vi "Exist Section.vi"(10 "sections":string[](array[string]), 11 "info data":string) -> (1 "exist":bool, 2 "after end of section":string, 3 "before end of section":string)   [LabVIEW 2013, in "infolib.lvlib"]
doc: "Checks if sections structure exists, if so divides string before the end of least significant section."
uses:
  infolib.lvlib
  <vilib>/regexp/Match Regular Expression.xnode
panel:
  out "regexp":string
  # "testing string: (put \"1\" and \"2\" into section names)"
  # "blfdablad\n#startsection:: 1\njfkdla\n#startsection:: 2\ngroup2group2\n\t  \t#endsection:: 2\njdfkls\n#endsection:: 1\njfdklajfkdl"
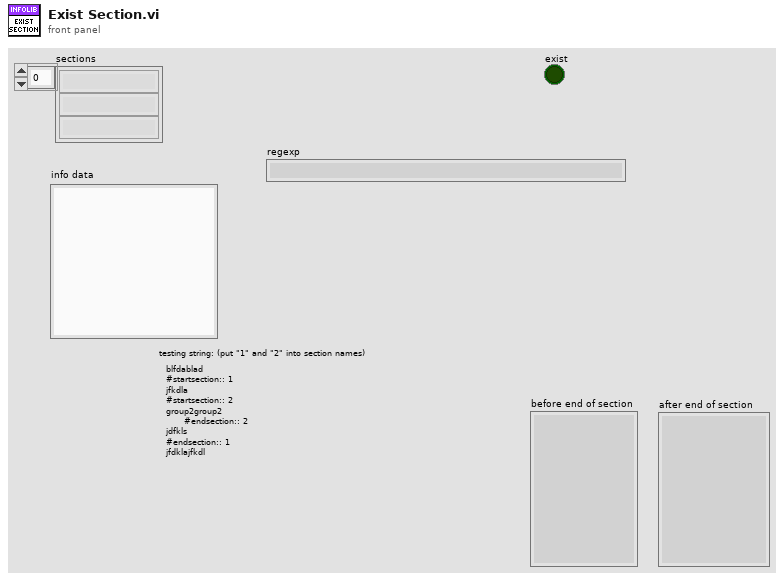
[diagram p1: front panel]
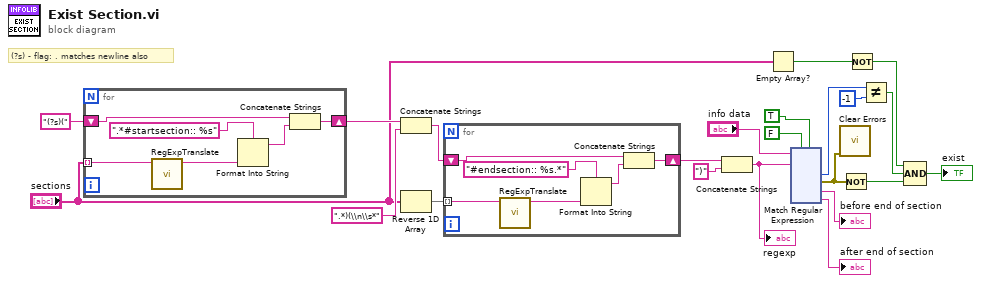
[diagram p0: block diagram]
diagram:
  # "(?s) - flag: . matches newline also"
  n1 = for {
    tunnel: "sections" -> [w24] mode=indexing
    shift-right: [w25] -> w17
    shift-left: "(?s)(" ("section name") -> [w26]
    n2 = call "RegExpTranslate.vi"("string"=w24) -> ("regexp safe string"=w23:string)  [unwired: 10 in]
    n3 = Format Into String(format string=".*#startsection:: %s", w23) -> (resulting string=w27:string)  [unwired: 2 in, 1 out]
    n4 = Concatenate Strings(w26, w27) -> (w25:string)
  }
  n5 = Concatenate Strings(w17, ".*)(\\n\\s*" ("string")) -> (w15:string)
  n6 = Reverse 1D Array(array="sections") -> (reversed array=w14:string[])
  n7 = for {
    shift-right: [w32] -> w11
    shift-left: w15 -> [w31]
    tunnel: w14 -> [w30] mode=indexing
    n8 = call "RegExpTranslate.vi"("string"=w30) -> ("regexp safe string"=w29:string)  [unwired: 10 in]
    n9 = Format Into String(format string="#endsection:: %s.*", w29) -> (resulting string=w33:string)  [unwired: 2 in, 1 out]
    n10 = Concatenate Strings(w31, w33) -> (w32:string)
  }
  n11 = Concatenate Strings(w11, ")" ("string")) -> (w10:string)
  "regexp" <- w10
  n12 = Empty Array?(array="sections") -> (empty?=w4:bool)
  n13 = xnode "Match Regular Expression"("input string"="info data", "regular expression"=w10, "ignore case? (F)"=FALSE, "multiline? (F)"=TRUE) -> ("offset past match"=w19:i32, "error out"=w1:errorcluster, "submatch 1"=→"before end of section":string, "submatch 2"=→"after end of section":string)  [unwired: 2 in, 3 out]
  n14 = call <vilib>:"Clear Errors.vi"("error in (no error)"=w1) -> ()  [unwired: 6 in, 1 out]
  n15 = Not(x=w1) -> (.not. x?=w2:bool)
  n16 = Not(x=w4) -> (.not. x?=w3:bool)
  n17 = Not Equal?(x=w19, y=-1 ("x")) -> (x != y?=w5:bool)
  n18 = Compound Arithmetic op=AND(w3, w5, w2) -> (→"exist":bool)
